vi "solar_misc Rendezvous Create.vi"(8 "error in (no error)":errorcluster, 9 "Create if not found? (T)":bool=TRUE, 10 "Size (0=Use Existing)":u32, 11 "Name":string) -> (0 "error out":errorcluster, 1 "Created New?":bool, 3 "Rendezvous":refnum<queue>)   [LabVIEW 2018]
doc: "This is a simplified version of NI's rendezvous create VI."
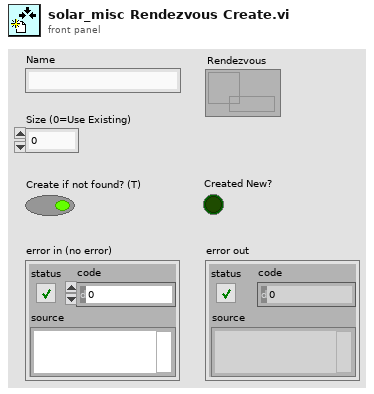
[diagram p1: front panel]
types:
  T1 = cluster{"Size":u32, "Rendezvous":refnum<queue>[]}
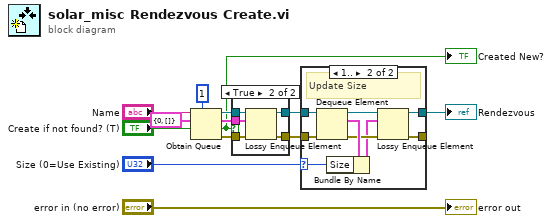
[diagram p0: block diagram]
diagram:
  w4 = T1 {"Size"=0, "Rendezvous"=[]} ("Rendezvous")
  n1 = Obtain Queue(max queue size (-1, unlimited)=1, name (unnamed)="Name", element data type=w4, create if not found? (T)="Create if not found? (T)") -> (queue out=w9:refnum<queue>, created new?=w2:bool, error out=w6:errorcluster)  [unwired: 1 in]
  "Created New?" <- w2
  n2 = case shown="True" w2 {
    tunnel: w9 -> [w14 w19]
    tunnel: [w14 w18] -> w7
    tunnel: w6 -> [w13 w17]
    tunnel: [w13 w16] -> w5
    tunnel: w4 -> [_ w15]
    frame False {
    }
    frame True {
      n3 = Lossy Enqueue Element(queue=w19, element=w15, error in (no error)=w17) -> (queue out=w18:refnum<queue>, error out=w16:errorcluster)  [unwired: 2 out]
    }
  }
  n4 = case shown="1.." "Size (0=Use Existing)" {
    selector: "Size (0=Use Existing)" -> [_ w27]
    tunnel: w7 -> [w21 w30]
    tunnel: w5 -> [w20 w29]
    tunnel: [w21 w23] -> w1
    tunnel: [w20 w22] -> _
    frame 0 {
    }
    frame 1.. {
      # "Update Size"
      n5 = Dequeue Element(queue=w30, error in (no error)=w29) -> (queue out=w26:refnum<queue>, element=w28:T1, error out=w25:errorcluster)  [unwired: 1 in, 1 out]
      n6 = Bundle By Name(cluster=w28, "Size"=w27) -> (w24:T1)
      n7 = Lossy Enqueue Element(queue=w26, element=w24, error in (no error)=w25) -> (queue out=w23:refnum<queue>, error out=w22:errorcluster)  [unwired: 2 out]
    }
  }
  "Rendezvous" <- w1
  "error out" <- "error in (no error)"
